vi "SR2000Test.vi"() -> ()   [LabVIEW 2014]
uses:
  controls/Data.ctl
panel:
  out "BarCodeRead":string
  out "Data Out":T1
  in  "Data In":T1
  # "日期"
  # "機種名稱"
  # "機種代號"
  # "商品條碼"
  # "台"
  # "OK"
  # "NG"
  # "台"
  # "總計"
  # "台"
  # "日期"
  # "機種名稱"
  # "機種代號"
  # "商品條碼"
  # "台"
  # "OK"
  # "NG"
  # "台"
  # "總計"
  # "台"
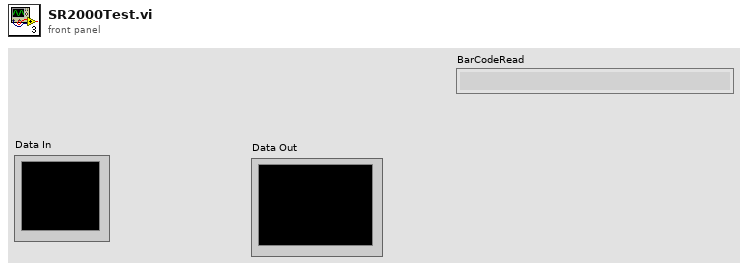
[diagram p1: front panel]
types:
  T1 = typedef "Data.ctl" = cluster{"Date":string, "BarCode1":string, "BarCode2":string, "BarCode3":string, "Message":string, "OK Count":u16, "NG Count":u16, "Total Count":u16, "ModelData":string[][], "OK&NG":bool, "COM1":refnum<visa-resource-name>, "COM2":refnum<visa-resource-name>, "IO":i32, "Time":u32, "TCP":refnum<k5>, "TCP 2":refnum<k5>}
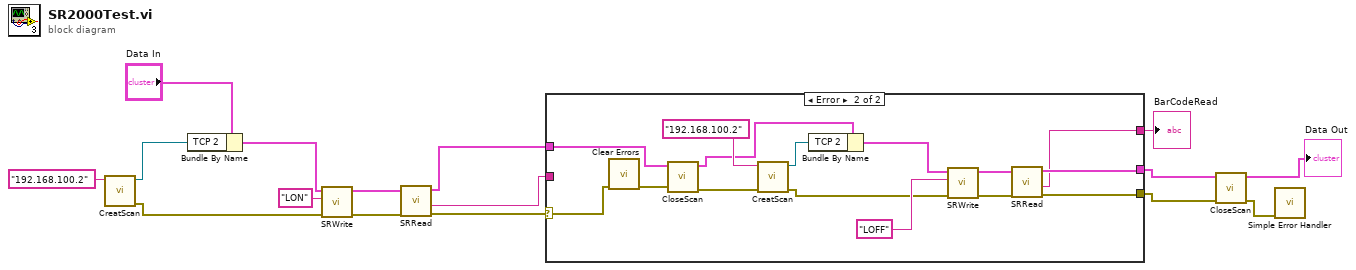
[diagram p0: block diagram]
diagram:
  n1 = call "CreatScan.vi"("address"="192.168.100.2") -> ("error out"=w9:errorcluster, "TCP Out"=w11:refnum<k5>)  [unwired: 8 in, 1 out]
  n2 = Bundle By Name(cluster="Data In", "TCP 2"=w11) -> (w10:T1)
  n3 = call "SRWrite.vi"("error in (no error)"=w9, "Command"="LON", "Data In"=w10) -> ("error out"=w15:errorcluster, "Data Out"=w16:T1)  [unwired: 7 in]
  n4 = call "SRRead.vi"("error in (no error)"=w15, "Data In"=w16) -> ("error out"=w8:errorcluster, "BarCodeRead"=w6:string, "Data Out"=w7:T1)  [unwired: 7 in]
  n5 = case shown="Error" w8 {
    selector: w8 -> [w17 w33]
    tunnel: w7 -> [w18 w30]
    tunnel: [w19 w20] -> w2
    tunnel: w6 -> [w19 _]
    tunnel: [w18 w23] -> w4
    tunnel: [w17 w21] -> w5
    frame No Error {
    }
    frame Error {
      n6 = call <vilib>:"Clear Errors.vi"("error in (no error)"=w33) -> ("error out"=w31:errorcluster)  [unwired: 5 in, 1 out]
      n7 = call "CloseScan.vi"("error in (no error)"=w31, "Data In"=w30) -> ("error out"=w28:errorcluster, "Data Out"=w29:T1)  [unwired: 8 in]
      n8 = call "CreatScan.vi"("error in (no error)"=w28, "address"="192.168.100.2") -> ("error out"=w25:errorcluster, "TCP Out"=w32:refnum<k5>)  [unwired: 7 in, 1 out]
      n9 = Bundle By Name(cluster=w29, "TCP 2"=w32) -> (w26:T1)
      n10 = call "SRWrite.vi"("error in (no error)"=w25, "Command"="LOFF", "Data In"=w26) -> ("error out"=w22:errorcluster, "Data Out"=w24:T1)  [unwired: 7 in]
      n11 = call "SRRead.vi"("error in (no error)"=w22, "Data In"=w24) -> ("error out"=w21:errorcluster, "BarCodeRead"=w20:string, "Data Out"=w23:T1)  [unwired: 7 in]
    }
  }
  "BarCodeRead" <- w2
  n12 = call "CloseScan.vi"("error in (no error)"=w5, "Data In"=w4) -> ("error out"=w1:errorcluster, "Data Out"=→"Data Out":T1)  [unwired: 8 in]
  n13 = call <vilib>:"Simple Error Handler.vi"("error in (no error)"=w1) -> ()  [unwired: 4 in, 5 out]
